vi "Manual-Auto.vi"() -> ()   [LabVIEW 2011]
panel:
  out "Auto/Manual":bool
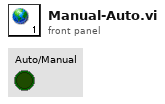
[diagram p1: front panel]
diagram:
